vi "CloseConnection.vi"(8 "error in (no error)":errorcluster, 11 "RS232 In":refnum<class "RS232.lvclass">) -> (0 "error out":errorcluster, 3 "RS232 Out":refnum<class "RS232.lvclass">)   [LabVIEW 2019, in "RS232.lvclass"]
uses:
  RS232.lvclass
  RS232.lvclass/RS232.ctl
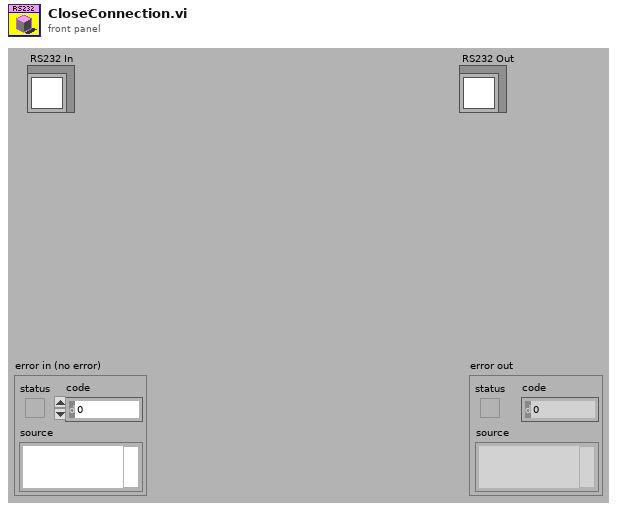
[diagram p1: front panel]
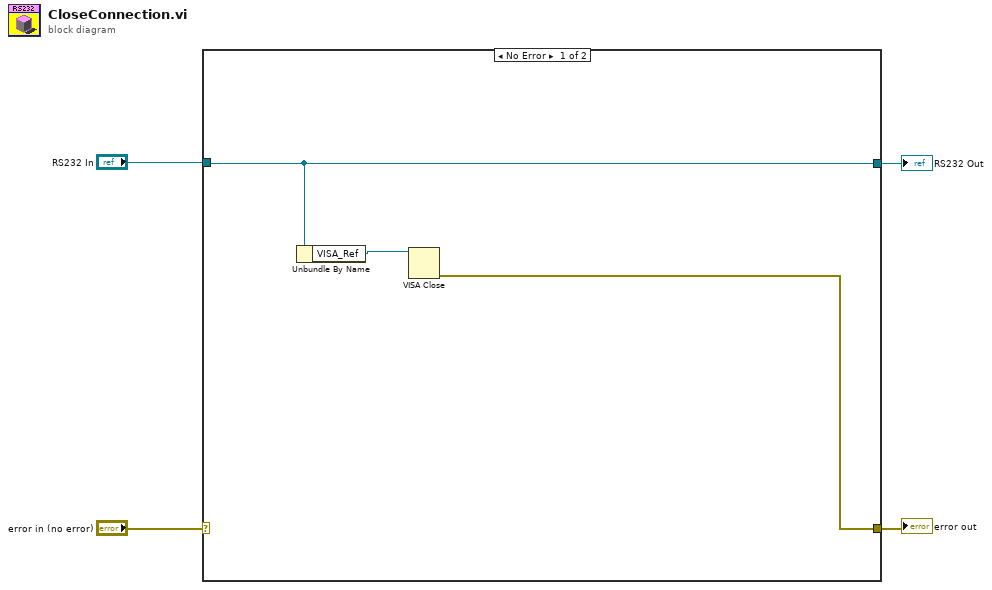
[diagram p0: block diagram]
diagram:
  n1 = case shown="No Error" "error in (no error)" {
    selector: "error in (no error)" -> [_ w9]
    tunnel: [w5 w9] -> w3
    tunnel: [w7 w8] -> w1
    tunnel: "RS232 In" -> [w7 w8]
    frame No Error {
      n2 = Unbundle By Name(w7) -> ("VISA_Ref"=w6:refnum<visa-resource-name>)
      n3 = VISA Close(VISA resource name=w6) -> (error out=w5:errorcluster)  [unwired: 1 in]
    }
    frame Error {
    }
  }
  "error out" <- w3
  "RS232 Out" <- w1
